vi "Load_RegDests.vi"(8 "error in (no error)":errorcluster, 11 "Class in":refnum<class "IB_MSI.lvclass">) -> (0 "error out":errorcluster, 3 "Class out":refnum<class "IB_MSI.lvclass">)   [LabVIEW 2020, in "IB_MSI.lvclass"]
uses:
  <vilib>/AppBuilder/IB_Classes/MSI/IB_MSI.lvclass
  <vilib>/AppBuilder/IB_Classes/MSI/IB_MSI.lvclass/IB_MSI.ctl
  <vilib>/AppBuilder/IB_Classes/Installer/Installer.lvclass
  <vilib>/AppBuilder/IB_Classes/RegDest/RegDest_User/IB_RegDest_User.lvclass
  <vilib>/AppBuilder/IB_Classes/RegDest/RegDest_Label/IB_RegDest_Label.lvclass
  <vilib>/AppBuilder/IB_Classes/RegDest/IB_RegDest.lvclass
  <resource>/Framework/Providers/Builds/Installer/CDK_sTypeDef_DirInfo.ctl
  e:/builds/penguin/labview/branches/2020/dev/dist/vi.lib/AppBuilder/IB_Classes/RegDest/IB_RegDest.lvclass
  e:/builds/penguin/labview/branches/2020/dev/dist/vi.lib/AppBuilder/IB_Classes/RegDest/RegDest_User/IB_RegDest_User.lvclass
  e:/builds/penguin/labview/branches/2020/dev/dist/vi.lib/AppBuilder/IB_Classes/Installer/Installer.lvclass
  e:/builds/penguin/labview/branches/2020/dev/dist/vi.lib/AppBuilder/IB_Classes/MSI/IB_MSI.lvclass
  e:/builds/penguin/labview/branches/2020/dev/dist/vi.lib/AppBuilder/IB_Classes/RegDest/RegDest_Label/IB_RegDest_Label.lvclass
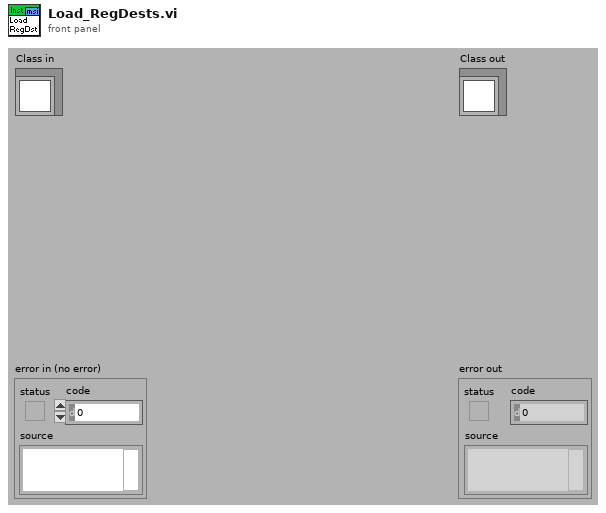
[diagram p1: front panel]
types:
  T1 = typedef "CDK_sTypeDef_DirInfo.ctl" = cluster{"ParentTag":string, "DirTag":string, "DirName":string, "Editable?":bool}
  T2 = typedef "IB_Installer.ctl" = cluster{"Destination":refnum<class "IB_Destination.lvclass">[], "Source":refnum<class "IB_Source.lvclass">[], "buildObject":T3, "defaultDir":string, "platform":string, "author":string, "productName":string, "buildSpecName":string, "hide":bool, "requireLVDevSys":bool, "autoIncrement":bool, "includeError":bool, "readmeID":string, "buildLocation":path, "readmePath":path, "mediaSize":u16, "language":T4, "productVersion":T5, "preview":bool, "programmatic":bool, "progressBarEvents":T6, "userLog_Path":path, "shortcutAddresses":T8[], "EXE_Install Address":string, "EXE_Uninstall Address":string, "additional NIPaths":refnum<class "Dest_NI_NIPath.lvclass">[], "web service itemIDs":string[], "installerName":string}
  T3 = typedef "ItemRef.ctl" = u64
  T4 = typedef "CDK_sTypeDef_Languages.ctl" = u16
  T5 = typedef "CDK_sTypeDef_ProductVersion.ctl" = cluster{"Major":u8, "Minor":u8, "Update":u16}
  T6 = typedef "provcom_ProgressBar_Events.ctl" = cluster{"newJob":refnum<user-event>, "newItem":refnum<user-event>, "errorMsg":T7, "cancel":refnum<user-event>}
  T7 = typedef "mxLvBuildError.ctl" = refnum<user-event>
  T8 = typedef "CDK_sTypeDef_ShortcutAddress.ctl" = cluster{"file":string, "shortcut":string}
  T9 = typedef "IB_RegDest.ctl" = cluster{"parentTag":string, "dirTag":string, "dirName":string, "unlock":bool, "path":string, "regData":refnum<class "IB_RegData.lvclass">[]}
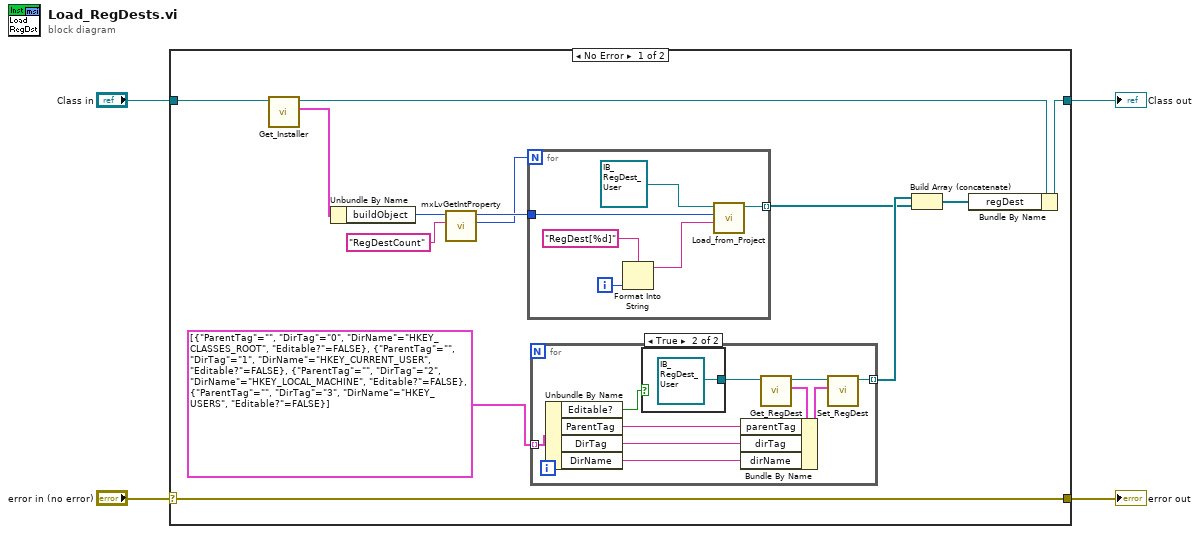
[diagram p0: block diagram]
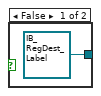
[diagram p2: hidden frame]
diagram:
  n1 = case shown="No Error" "error in (no error)" {
    selector: "error in (no error)" -> [w9 w37]
    tunnel: [w9 w37] -> w3
    tunnel: [w13 w36] -> w1
    tunnel: "Class in" -> [w12 w36]
    frame No Error {
      n2 = call <vilib>:"Get_Installer.vi"("Installer in"=w12) -> ("data"=w10:T2, "Installer out"=w11:refnum<class "IB_MSI.lvclass">)  [unwired: 1 in, 8 out]
      n3 = Unbundle By Name(w10) -> ("buildObject"=w16:T3)
      n4 = call <resource>:"mxLvGetIntProperty.vi"("Tag"="RegDestCount", "Item"=w16) -> ("Value"=w14:i32, "Item"=w15:T3)  [unwired: 1 in, 7 out]
      n5 = for {
        N: w14 -> [_]
        tunnel: w15 -> [w32]
        tunnel: [w35] -> w7 mode=indexing
        i -> [w33]
        n6 = Format Into String(format string="RegDest[%d]", w33) -> (resulting string=w30:string)  [unwired: 2 in, 1 out]
        n7 = call-dynamic "Load_from_Project.vi"("index"=w30, "buildObject"=w32, "IB_RegDest in"=refnum<class "IB_RegDest_User.lvclass"> refnum ("IB_RegDest_User.lvclass")) -> ("IB_RegDest out"=w35:refnum<class "IB_RegDest_User.lvclass">)  [unwired: 1 in, 7 out]
      }
      n8 = for {
        tunnel: T1[] [{"ParentTag"="", "DirTag"="0", "DirName"="HKEY_CLASSES_ROOT", "Editable?"=FALSE}, {"ParentTag"="", "DirTag"="1", "DirName"="HKEY_CURRENT_USER", "Editable?"=FALSE}, {"ParentTag"="", "DirTag"="2", "DirName"="HKEY_LOCAL_MACHINE", "Editable?"=FALSE}, {"ParentTag"="", "DirTag"="3", "DirName"="HKEY_USERS", "Editable?"=FALSE}] ("Array") -> [w27] mode=indexing
        tunnel: [w19] -> w8 mode=indexing
        n9 = Unbundle By Name(w27) -> ("Editable?"=w18:bool, "ParentTag"=w22:string, "DirTag"=w21:string, "DirName"=w20:string)
        n10 = case shown="True" w18 {
          tunnel: [refnum<class "IB_RegDest_Label.lvclass"> refnum ("IB_RegDest_Label.lvclass") refnum<class "IB_RegDest_User.lvclass"> refnum ("IB_RegDest_User.lvclass")] -> w25
          frame False {
          }
          frame True {
          }
        }
        n11 = call <vilib>:"Get_RegDest.vi"("Class in"=w25) -> ("data"=w24:T9, "Class out"=w26:refnum<class "IB_RegDest.lvclass">)  [unwired: 1 in, 8 out]
        n12 = Bundle By Name(cluster=w24, "parentTag"=w22, "dirTag"=w21, "dirName"=w20) -> (w23:T9)
        n13 = call <vilib>:"Set_RegDest.vi"("data"=w23, "Class in"=w26) -> ("Class out"=w19:refnum<class "IB_RegDest.lvclass">)  [unwired: 1 in, 8 out]
      }
      n14 = Build Array (concatenate)(w8, w7) -> (w6:refnum<class "IB_RegDest.lvclass">[])
      n15 = Bundle By Name(cluster=w11, "regDest"=w6) -> (w13:refnum<class "IB_MSI.lvclass">)
    }
    frame Error {
    }
  }
  "error out" <- w3
  "Class out" <- w1
